vi "split can read data.vi"(6 "CAN DATA 3":T1[](array[typedef]) {"Data" format="%.0x"; "ArbitrationId" format="%.0x"; "Timestamp" format="%<%I:%M:%S%3u %p\n%m/%d/%Y>T"}, 8 "error constant":errorcluster, 9 "101 array":T1[](array[typedef]) {"Data" format="%.0x"; "ArbitrationId" format="%.0x"; "Timestamp" format="%<%I:%M:%S%3u %p\n%m/%d/%Y>T"}, 10 "Array":u32[][](array[numeric]) format="%x", 11 "CAN DATA":T1[](array[typedef]) {"Data" format="%.0x"; "ArbitrationId" format="%.0x"; "Timestamp" format="%<%I:%M:%S%3u %p\n%m/%d/%Y>T"}) -> (0 "error out":errorcluster, 1 "element":T1 {"Data" format="%.0x"; "ArbitrationId" format="%.0x"; "Timestamp" format="%<%I:%M:%S%3u %p\n%m/%d/%Y>T"}, 2 "101 Array":T1[](array[typedef]) {"Data" format="%.0x"; "ArbitrationId" format="%.0x"; "Timestamp" format="%<%I:%M:%S%3u %p\n%m/%d/%Y>T"}, 3 "sorted 2D array":u32[][](array[numeric]) format="%x", 4 "CAN DATA 2":T1[](array[typedef]) {"Data" format="%.0x"; "ArbitrationId" format="%.0x"; "Timestamp" format="%<%I:%M:%S%3u %p\n%m/%d/%Y>T"})   [LabVIEW 2017]
uses:
  <vilib>/nican/nican.llb/CanFrameTimed.ctl
  62b90f59-21b7-4b33-8261-6c9e1ca4df07.vi
  <vilib>/Array/Sort 2D Array - Pop Stack.vi
  <vilib>/Array/Sort 2D Array - Push Stack.vi
panel:
  in  "CAN TABLE":string[][](array[string])
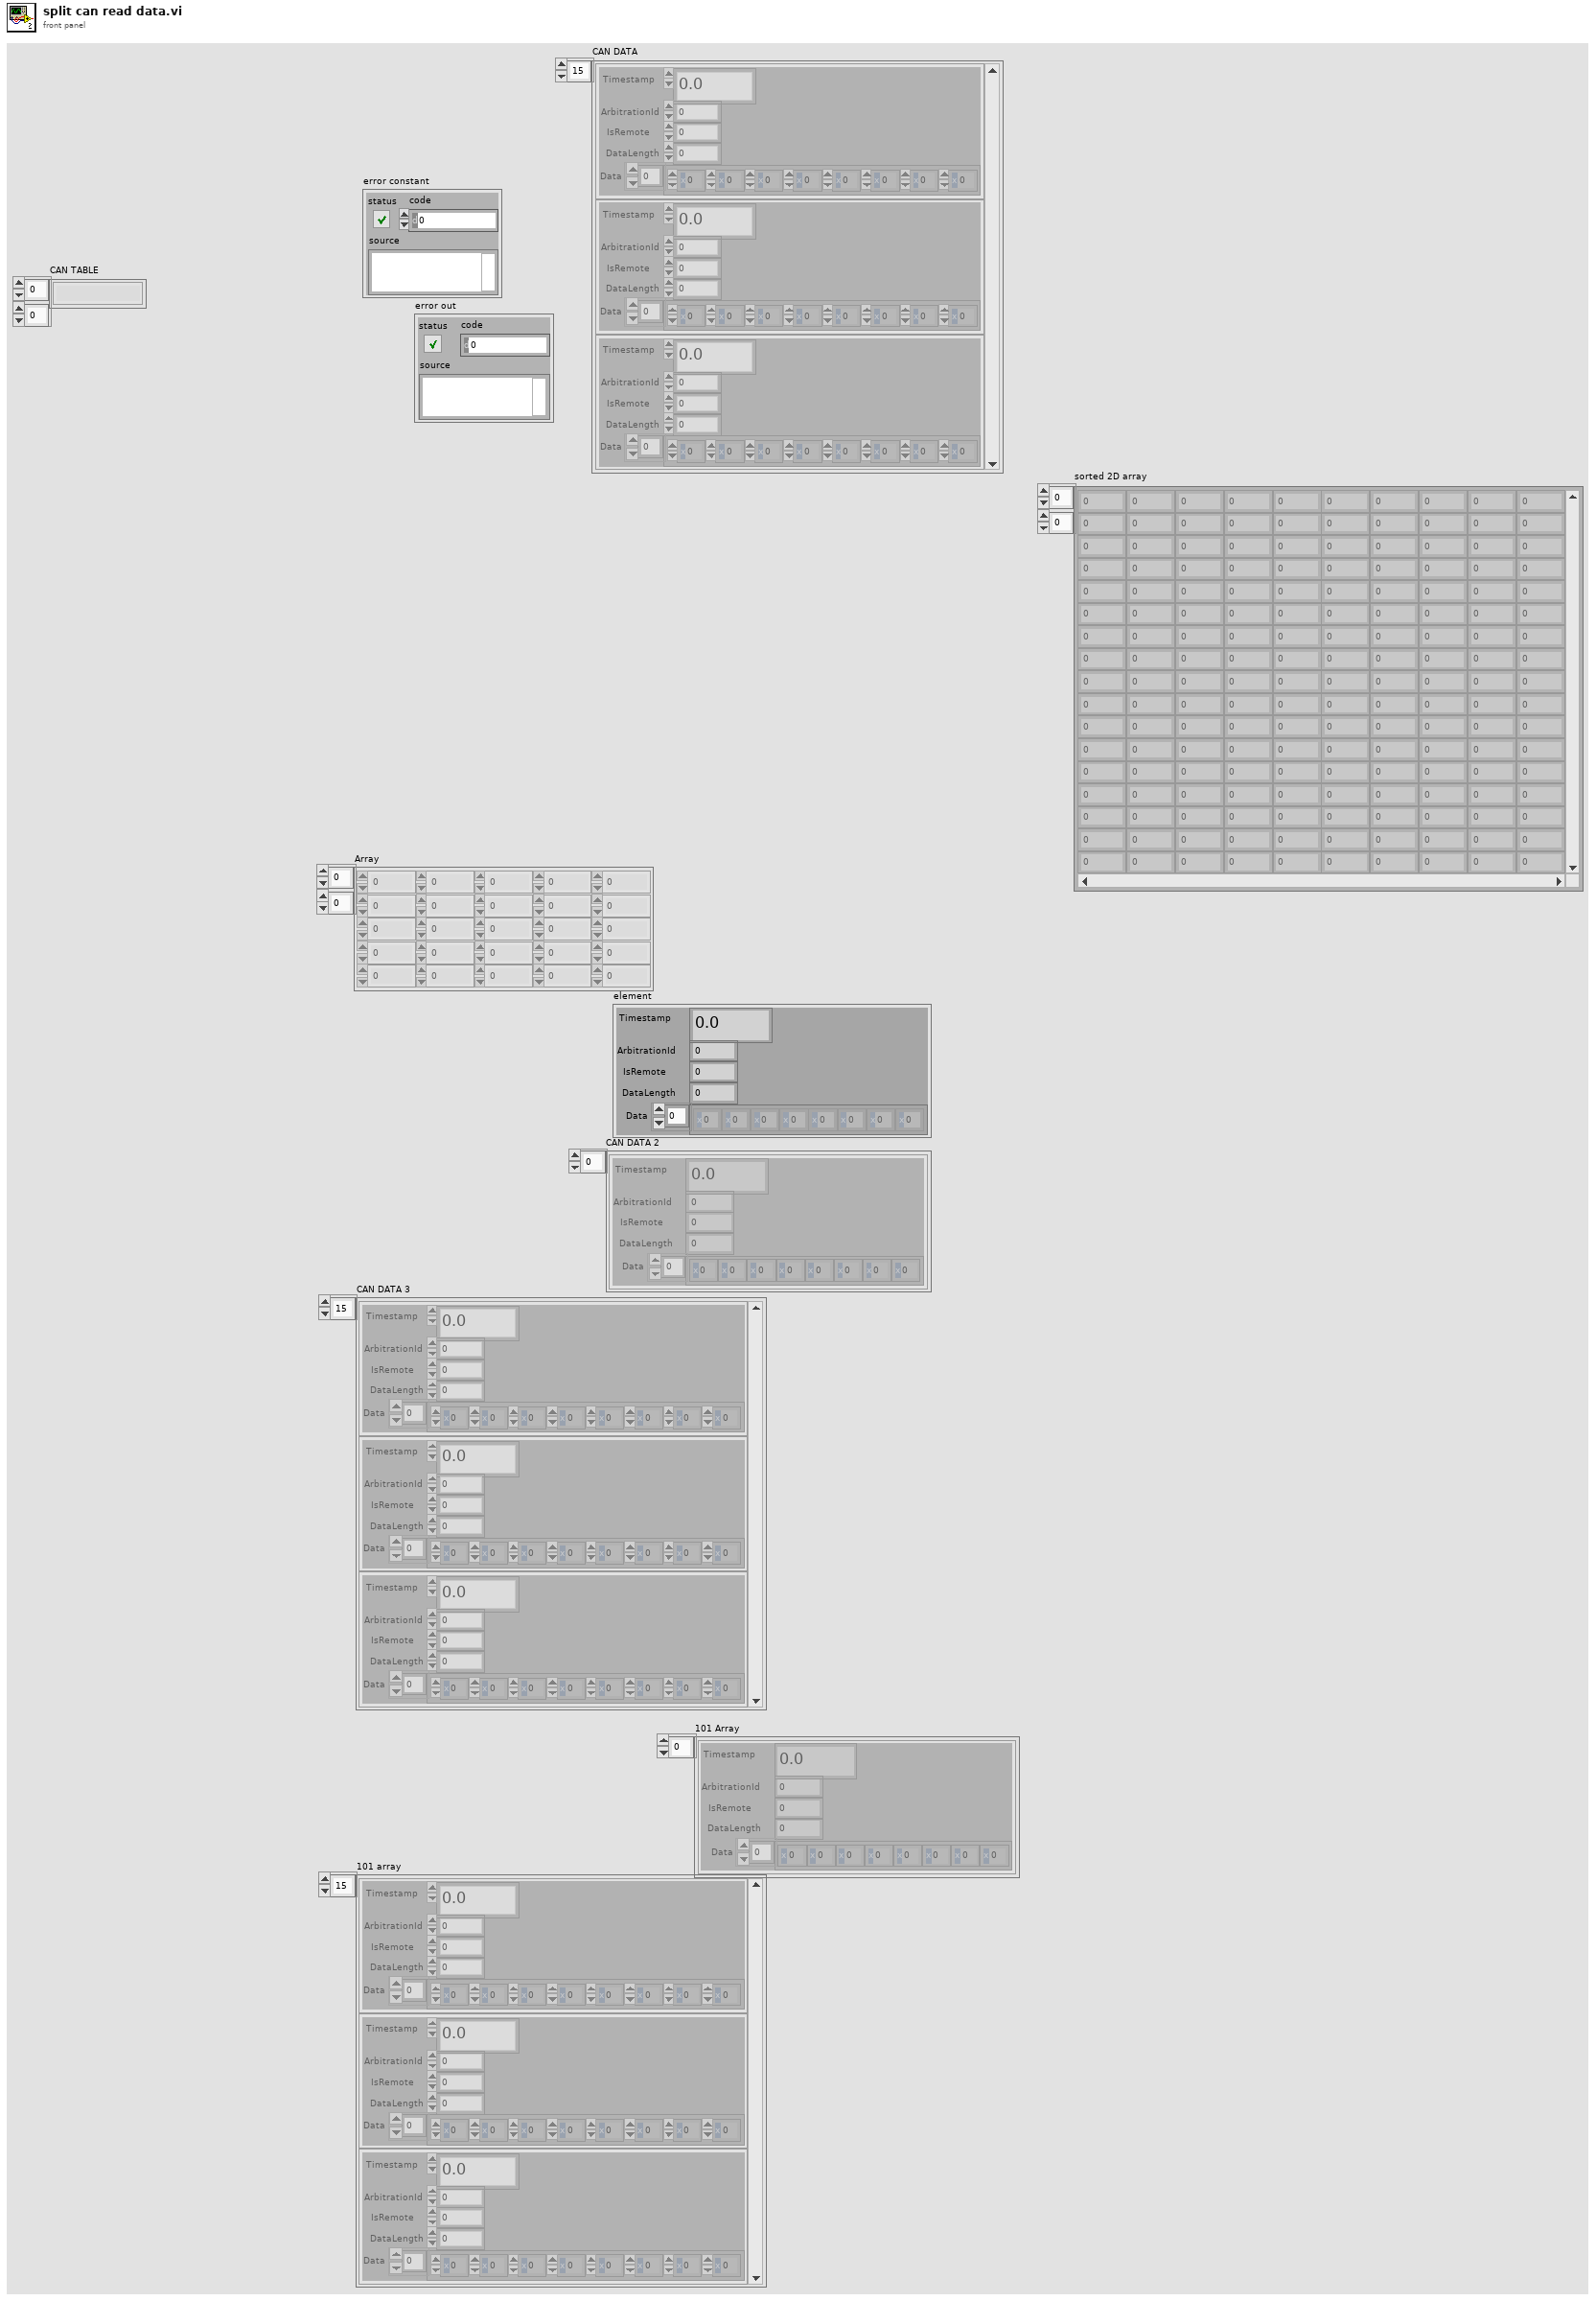
[diagram p1: front panel]
types:
  T1 = typedef "CanFrameTimed.ctl" = cluster{"Timestamp":dbl, "ArbitrationId":u32, "IsRemote":u8, "DataLength":u8, "Data":u8[]}
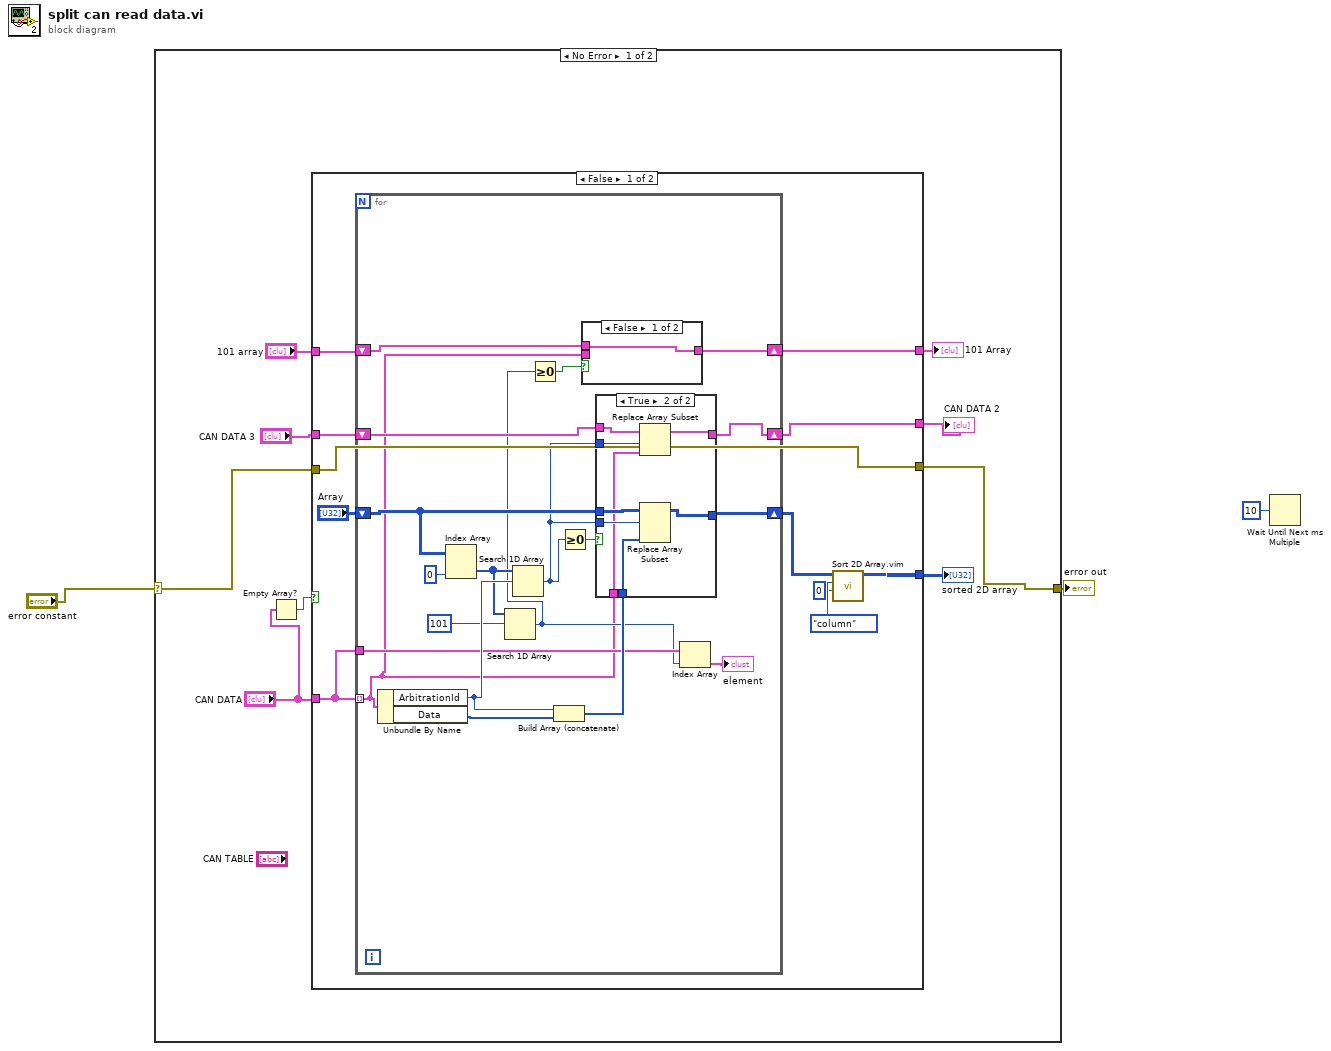
[diagram p0: block diagram]
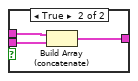
[diagram p2: hidden frame]
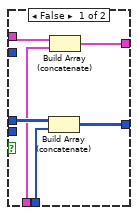
[diagram p3: hidden frame]
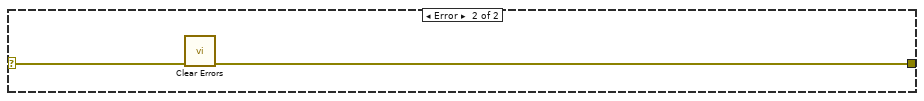
[diagram p5: hidden frame]
diagram:
  n1 = case shown="No Error" "error constant" {
    selector: "error constant" -> [w10 w65]
    tunnel: [w9 w64] -> w2
    frame No Error {
      n2 = Empty Array?(array="CAN DATA") -> (empty?=w11:bool)
      n3 = case shown="False" w11 {
        tunnel: [w20 _] -> w12
        tunnel: "CAN DATA" -> [w17 _]
        tunnel: [w18 w63] -> w9
        tunnel: w10 -> [w18 w63]
        tunnel: [w16 w62] -> w8
        tunnel: "CAN DATA 3" -> [w15 w62]
        tunnel: [w14 w61] -> w5
        tunnel: "101 array" -> [w13 w61]
        frame False {
          n4 = for {
            tunnel: w17 -> [w28] mode=indexing
            shift-right: [w40] -> w23
            shift-left: "Array" -> [w35]
            tunnel: w17 -> [w34]
            shift-right: [w31] -> w16
            shift-left: w15 -> [w32]
            shift-right: [w27] -> w14
            shift-left: w13 -> [w26]
            n5 = Unbundle By Name(w28) -> ("ArbitrationId"=w38:u32, "Data"=w42:u8[])
            n6 = Index Array(array=w35, index (col)=0 ("disabled index (col)")) -> (element=w36:u32[])  [unwired: 1 in]
            n7 = Search 1D Array(1D array=w36, element=u32 101 ("ArbitrationId")) -> (index of element=w30:i32)  [unwired: 1 in]
            n8 = Search 1D Array(1D array=w36, element=w38) -> (index of element=w25:i32)  [unwired: 1 in]
            n9 = Greater Or Equal To 0?(x=w30) -> (x >= 0?=w29:bool)
            n10 = Build Array (concatenate)(w38, w42) -> (w41:u32[])
            n11 = Greater Or Equal To 0?(x=w25) -> (x >= 0?=w24:bool)
            n12 = case shown="False" w29 {
              tunnel: w28 -> [_ w46]
              tunnel: [w43 w45] -> w27
              tunnel: w26 -> [w43 w44]
              frame False {
              }
              frame True {
                n13 = Build Array (concatenate)(w44, w46) -> (w45:T1[])
              }
            }
            n14 = case shown="True" w24 {
              tunnel: w35 -> [w52 w60]
              tunnel: w41 -> [w51 w59]
              tunnel: w25 -> [_ w58]
              tunnel: [w50 w57] -> w40
              tunnel: w32 -> [w49 w56]
              tunnel: [w48 w55] -> w31
              tunnel: w28 -> [w47 w53]
              tunnel: w25 -> [_ w54]
              frame False {
                n15 = Build Array (concatenate)(w52, w51) -> (w50:u32[][])
                n16 = Build Array (concatenate)(w49, w47) -> (w48:T1[])
              }
              frame True {
                n17 = Replace Array Subset(array=w56, new element=w53, index=w54) -> (w55:T1[])
                n18 = Replace Array Subset(array=w60, new element=w59, index (row)=w58) -> (w57:u32[][])  [unwired: 1 in]
              }
            }
            n19 = Index Array(array=w34, index=w30) -> (element=→"element":T1)
          }
          n20 = call "Sort 2D Array.vim"("index"=0, "dimension to index (column)"=enum16{"column", "row"}."column", "2D array"=w23) -> ("sorted 2D array"=w20:u32[][])  [unwired: 7 in, 1 out]
        }
        frame True {
        }
      }
      "sorted 2D array" <- w12
      "CAN DATA 2" <- w8
      "101 Array" <- w5
    }
    frame Error {
      n21 = call <vilib>:"Clear Errors.vi"("error in (no error)"=w65) -> ("error out"=w64:errorcluster)  [unwired: 5 in, 1 out]
    }
  }
  "error out" <- w2
  n22 = Wait Until Next ms Multiple(millisecond multiple=u32 10) -> ()  [unwired: 1 out]
